vi "get Textures And Hotspots.vi"(11 "Deployable in":refnum<class "Deployable.lvclass">) -> (2 "Hotspots":refnum<class "Vector 2D.lvclass">[](array[class]), 3 "Textures":string[](array[string]))   [LabVIEW 2021, in "Deployable.lvclass"]
uses:
  Deployable.lvclass
  Vector 2D/Vector 2D.lvclass
  Deployable.lvclass/Deployable.ctl
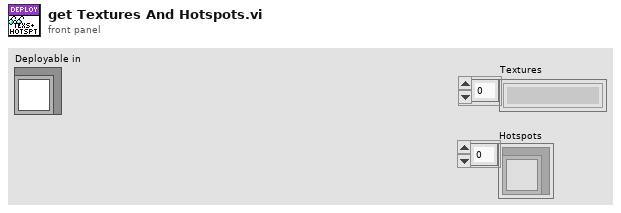
[diagram p1: front panel]
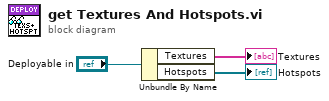
[diagram p0: block diagram]
diagram:
  n1 = Unbundle By Name("Deployable in") -> ("Textures"=→"Textures":string[], "Hotspots"=→"Hotspots":refnum<class "Vector 2D.lvclass">[])
